vi "Play Editor.vi"() -> ()   [LabVIEW 2015]
uses:
  Autonomous VIs/Autonomous Exec/Autonomous Play Definition.ctl
  Autonomous VIs/Autonomous Commands/Autonomous Command Names.ctl
  <vilib>/FTP/NI_FTP.lvlib
panel:
  in  "Connect\nto Robot":bool
  in  "Reload Folder":bool
  out "Error \nSending \nFiles":errorcluster
  out "Error \nRetrieving \nFiles":errorcluster
  in  "Empty Play Definition":T1 caption="Play"
  in  "Robot IP Address":string(combo)="10.xx.yy.2"
  in  "Download Plays":bool
  in  "Connected to Robot":bool
  in  "Send Plays":bool
  out "Create Play Error":errorcluster
  out "Play Read Error":errorcluster
  in  "Static Form":bool
  out "Commit Play Error":errorcluster
  in  "Current File Refnum":refnum<file>
  in  "Is a File":bool
  in  "Commit Play Changes":bool
  in  "Auto Directory":path
  in  "Finish":bool
  in  "Current Directory":path
  in  "Create New Play":bool
  in  "Play Selector Box":string(combo)
  in  "Play Currently Open":T1 caption="Play"
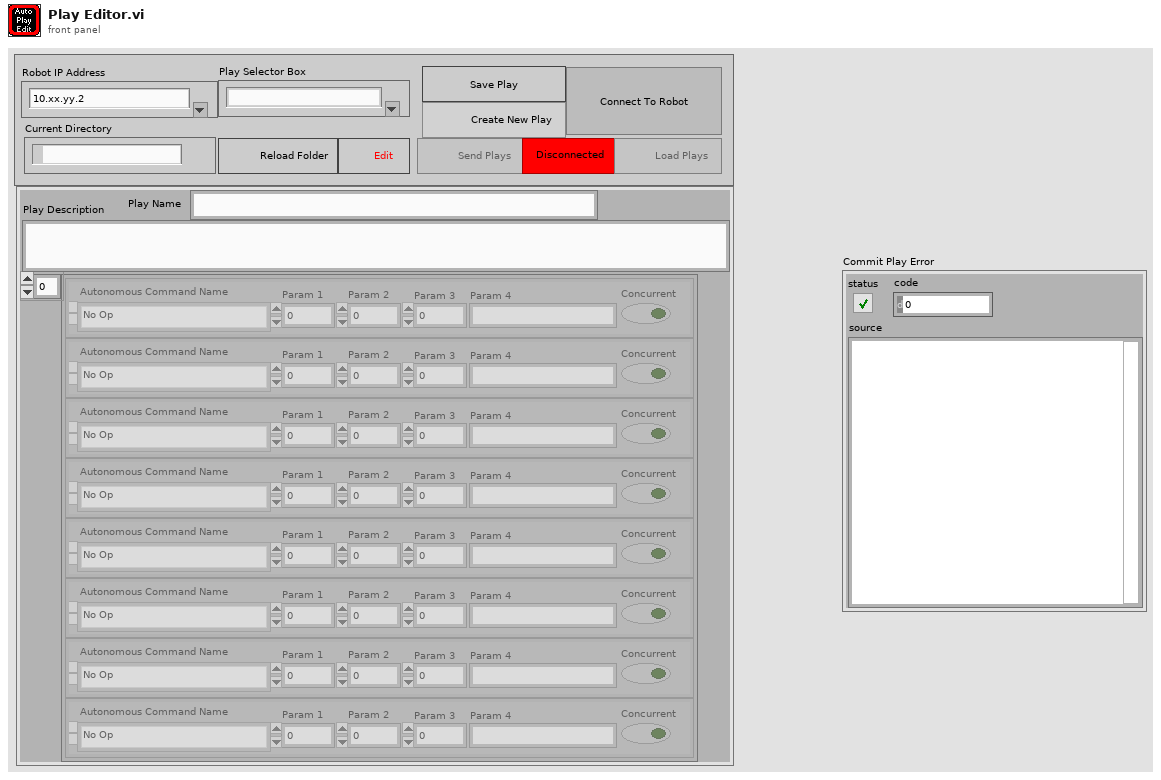
[diagram p1: front panel]
types:
  T1 = typedef "Autonomous Play Definition.ctl" = cluster{"Play Name":string, "Command List":cluster{"Param 1":dbl, "Param 2":dbl, "Autonomous Command Name":T2, "Concurrent":bool, "Param 3":dbl, "Param 4":string}[], "Play Description":string}
  T2 = typedef "Autonomous Command Names.ctl" = enum16{"No Op", "Drive Time", "Run Motion Profile", "Turn to Heading", "Turn To Target", "Cross Defense", "Fire", "Wait", "Reset Gyro", "Grabber Setpoints", "Manual Grabber", "Roller", "Autorange Command", "Reposition"}
  T3 = typedef "NI_FTP.lvlib/FTP Session.ctl" = refnum<k5>
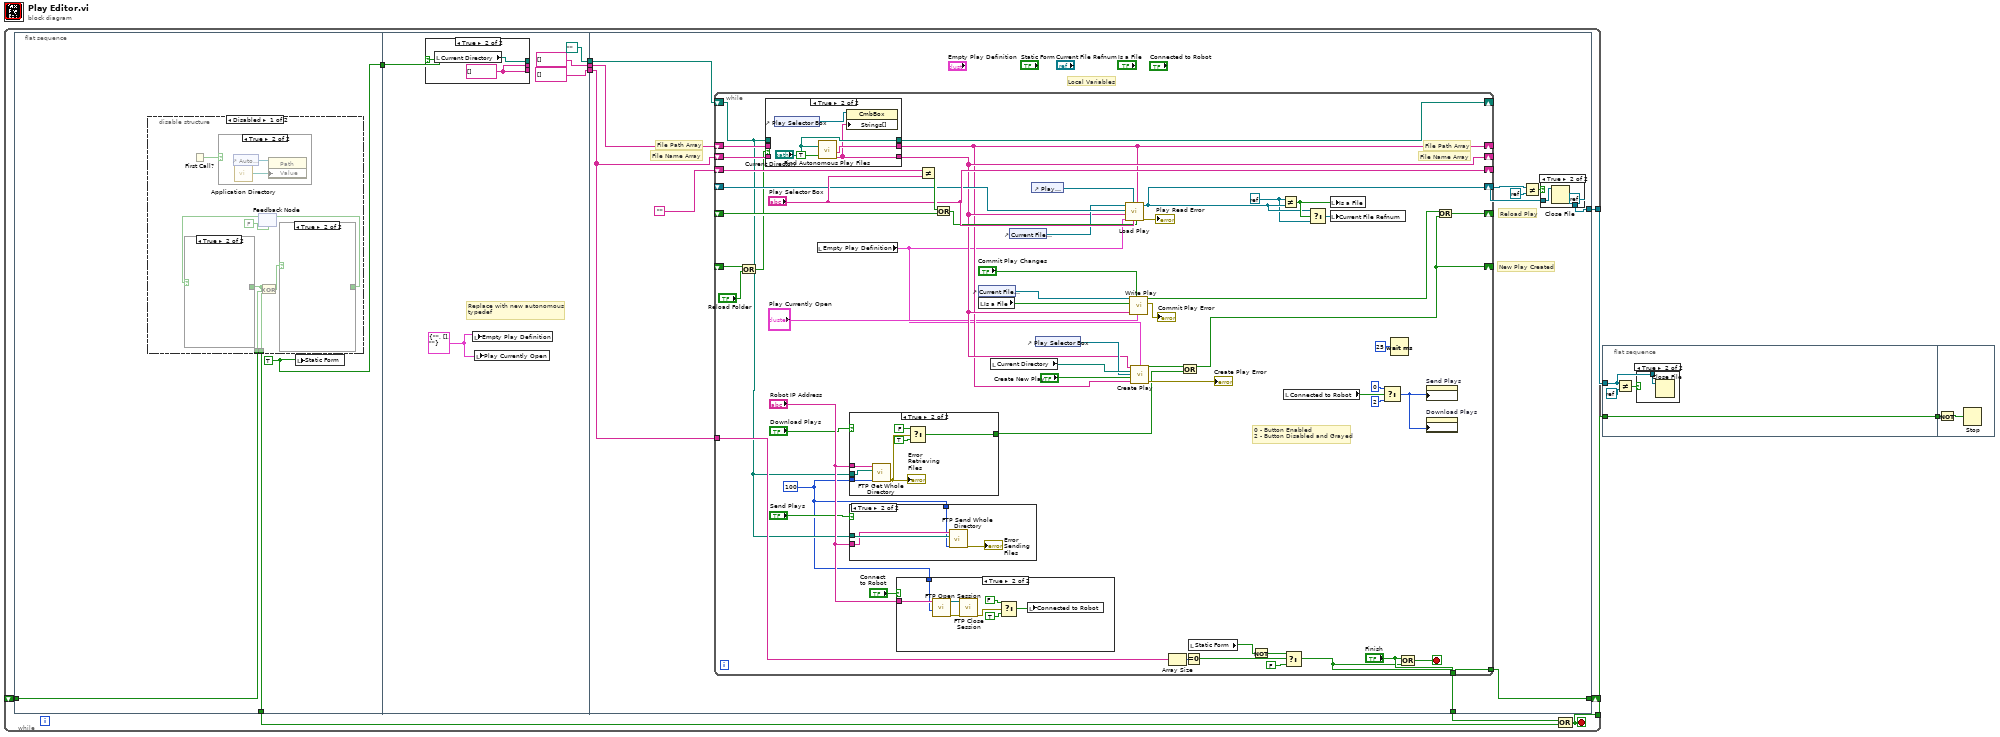
[diagram p0: block diagram]
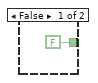
[diagram p3: hidden frame]
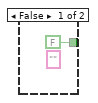
[diagram p4: hidden frame]
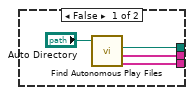
[diagram p7: hidden frame]
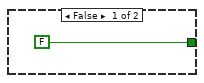
[diagram p11: hidden frame]
diagram:
  n1 = while {
    shift-right: [w10] -> _
    shift-left: _ -> [w9]
    tunnel: [w7] -> w2
    tunnel: [w6] -> w1
    stop <- w7 stop-if-true
    n2 = flat-sequence {
      tunnel: [w15] -> w8
      tunnel: w9 -> [w16]
      tunnel: [w14] -> w4
      tunnel: [string[] [] ("Filepath Array")] -> w13
      tunnel: [path "" ("Current Directory")] -> w12
      tunnel: [string[] [] ("Filepath Array")] -> w5
      tunnel: w4 -> [w32]
      tunnel: w13 -> [w40]
      tunnel: w12 -> [w39]
      tunnel: [w47] -> w11
      tunnel: [w44] -> w10
      tunnel: [w41] -> w6
      tunnel: w5 -> [w42]
      frame #0 {
        w14 = TRUE ("Static Form")
        n3 = disable-structure shown="Disabled" {
          disable-tunnel: w16 -> [w22 _]
          disable-tunnel: [w17 _] -> w15
          frame Disabled {
            n4 = First Call?() -> (First Call?: T/F=w23:bool)
            n5 = case shown="True" w23 {
              frame False {
              }
              frame True {
                n6 = control-ref of="Auto Directory"() -> (w27:refnum<vi>)
                n7 = call <vilib>:"Application Directory.vi"() -> ("Application Directory"=w26:path)
                n8 = property class="Path"(reference=w27, "Value"=w26) -> ()  [unwired: 1 in, 2 out]
              }
            }
            n9 = feedback #1(FALSE ("OK")) -> (w19:bool)
            n10 = case shown="True" w19 {
              tunnel: [FALSE ("No") _] -> w17
              frame False {
              }
              frame True {
              }
            }
            n11 = Exclusive Or(1:w22, 2:w17) -> (0:w21:bool)
            n12 = case shown="True" w21 {
              tunnel: [FALSE ("OK") _] -> w20
              frame False {
                (unwired) "" ("Full Directory")
              }
              frame True {
              }
            }
            n13 = feedback-in #1(w20) -> ()
          }
          frame Enabled {
          }
        }
        n14 = local write "Static Form"(w14) -> ()
      }
      frame #1 {
        w31 = T1 {"Play Name"="", "Command List"=[], "Play Description"=""} ("Play 1")
        # "Replace with new autonomous\ntypedef"
        n15 = case shown="True" w32 {
          tunnel: [w35 w37] -> _
          tunnel: [w34 w38] -> _
          tunnel: [w33 w38] -> _
          frame False {
            n16 = call "Find Autonomous Play Files.vi"("Application Directory"="Auto Directory") -> ("Application Directory"=w35:path, "Filepath Array"=w33:string[], "filename array"=w34:string[])  [unwired: 2 in, 1 out]
          }
          frame True {
            w38 = string[] [] ("Filepath Array")
            n17 = local read "Current Directory"() -> (w37:path)
          }
        }
        n18 = local write "Empty Play Definition"(w31) -> ()
        n19 = local write "Play Currently Open"(w31) -> ()
      }
      frame #2 {
        # "Local Variables"
        # "File Path Array"
        # "File Name Array"
        # "New Play Created"
        # "Reload Play"
        n20 = while {
          shift-right: ["Play Selector Box"] -> _
          shift-left: "" -> [w107]
          shift-right: [w98] -> w43
          shift-left: _ -> [w104]
          shift-right: [w82] -> _
          shift-left: _ -> [w94]
          tunnel: w40 -> [w102]
          tunnel: ["Finish"] -> w47
          tunnel: [w87] -> w44
          shift-right: [w60] -> _
          shift-left: _ -> [w57]
          shift-right: [w72] -> _
          shift-left: w42 -> [w84]
          shift-right: [w73] -> _
          shift-left: w40 -> [w83]
          shift-right: [w55] -> _
          shift-left: w39 -> [w54]
          stop <- w103 stop-if-true
          w53 = 100 ("timeout ms (60000)")
          w96 = refnum<k0> refnum
          # "0 - Button Enabled\n2 - Button Disabled and Grayed"
          # "File Path Array"
          # "File Name Array"
          n21 = Or(x=w57, y="Reload Folder") -> (x .or. y?=w58:bool)
          n22 = case shown="True" w58 {
            tunnel: [w130 w135] -> w72
            tunnel: [w129 w131] -> w73
            tunnel: w84 -> [w130 _]
            tunnel: w83 -> [w129 _]
            tunnel: w54 -> [w128 _]
            tunnel: [w128 "Current Directory"] -> w55
            frame False {
            }
            frame True {
              n23 = control-ref of="Play Selector Box"() -> (w132:refnum<vi>)
              n24 = call "Find Autonomous Play Files.vi"("Application Directory"="Current Directory", "Do not include file\nsuffix"=TRUE ("Do not include\nstring ending")) -> ("Filepath Array"=w135:string[], "filename array"=w131:string[])  [unwired: 1 in, 2 out]
              n25 = property class="CmbBox"(reference=w132, "Strings[]"=w131) -> ()  [unwired: 1 in, 2 out]
            }
          }
          n26 = local read "Empty Play Definition"() -> (w64:T1)
          n27 = case shown="True" "Download Plays" {
            tunnel: w54 -> [_ w127]
            tunnel: "Robot IP Address" -> [_ w126]
            tunnel: [FALSE ("Load New Play") w122] -> w59
            tunnel: w53 -> [_ w121]
            frame False {
            }
            frame True {
              n28 = call "FTP Get Whole Directory.vi"("timeout ms (60000)"=w121, "Local Folder of Autonomous Plays"=w127, "host"=w126) -> ("error out"=w125:errorcluster)  [unwired: 8 in]
              "Error \nRetrieving \nFiles" <- w125
              n29 = Select(t=FALSE, s=w125, f=TRUE ("Load New Play")) -> (s? t:f=w122:bool)
            }
          }
          n30 = case shown="True" "Send Plays" {
            tunnel: w54 -> [_ w119]
            tunnel: "Robot IP Address" -> [_ w118]
            tunnel: w53 -> [_ w116]
            frame False {
            }
            frame True {
              n31 = call "FTP Send Whole Directory.vi"("timeout ms (60000)"=w116, "Local Folder of Autonomous Plays"=w119, "host"=w118) -> ("error out"=→"Error \nSending \nFiles":errorcluster)  [unwired: 8 in]
            }
          }
          n32 = case shown="True" "Connect\nto Robot" {
            tunnel: "Robot IP Address" -> [_ w115]
            tunnel: w53 -> [_ w108]
            frame False {
            }
            frame True {
              n33 = call <vilib>:"FTP Open Session.vi"("timeout ms (60000)"=w108, "address"=w115) -> ("error out"=w113:errorcluster, "ftp session"=w114:T3)  [unwired: 6 in, 2 out]
              n34 = call <vilib>:"FTP Close Session.vi"("error in (no error)"=w113, "ftp session"=w114) -> ("error out"=w112:errorcluster)  [unwired: 6 in, 3 out]
              n35 = Select(t=FALSE, s=w112, f=TRUE) -> (s? t:f=w109:bool)
              n36 = local write "Connected to Robot"(w109) -> ()
            }
          }
          n37 = Not Equal?(x=w107, y="Play Selector Box") -> (x != y?=w106:bool)
          n38 = Or(x=w106, y=w94) -> (x .or. y?=w90:bool)
          n39 = control-ref of="Current File Refnum"() -> (w77:refnum<vi>)
          n40 = local read "Is a File"() -> (w78:bool)
          n41 = local read "Current Directory"() -> (w76:path)
          n42 = control-ref of="Current File Refnum"() -> (w80:refnum<vi>)
          n43 = control-ref of="Play Currently Open"() -> (w63:refnum<vi>)
          n44 = control-ref of="Play Selector Box"() -> (w75:refnum<vi>)
          n45 = call "Load Play.vi"("Load Play"=w90, "Filepath Array"=w72, "Play Selector Box"="Play Selector Box", "Play Currently Open Property Reference"=w63, "Empty Play Definition"=w64, "filename array"=w73, "Previous Iteration \nFile Refnum"=w104, "Current File Refnum"=w80) -> ("Read file error"=→"Play Read Error":errorcluster, "Output File Refnum"=w98:refnum<file>)  [unwired: 2 in]
          n46 = call "Write Play.vi"("Current Selected Play"="Play Currently Open", "Commit Play Changes"="Commit Play Changes", "filename array"=w73, "Is a File"=w78, "File Refnum"=w77) -> ("File Write Error"=→"Commit Play Error":errorcluster, "Not Cancelled\nLoad File"=w95:bool)  [unwired: 5 in]
          n47 = call "Create Play.vi"("Filename Array in"=w73, "Empty Play Definition"=w64, "Application Directory"=w76, "Play Selection Box Property Reference"=w75, "Create New Play"="Create New Play", "Filepath Array in"=w72) -> ("Load New Play"=w81:bool, "error out"=→"Create Play Error":errorcluster)  [unwired: 6 in, 2 out]
          n48 = Array Size(array=w102) -> (size(s)=w101:i32)
          n49 = Or(x=w81, y=w59) -> (x .or. y?=w60:bool)
          n50 = Equal To 0?(x=w101) -> (x = 0?=w89:bool)
          n51 = local read "Static Form"() -> (w88:bool)
          n52 = Not(x=w88) -> (.not. x?=w86:bool)
          n53 = Not Equal?(x=w96, y=w98) -> (x != y?=w99:bool)
          n54 = local read "Connected to Robot"() -> (w68:bool)
          n55 = Select(t=w86, s=w89, f=FALSE) -> (s? t:f=w87:bool)
          n56 = Select(t=w98, s=w99, f=w96) -> (s? t:f=w97:refnum<file>)
          n57 = local write "Is a File"(w99) -> ()
          n58 = local write "Current File Refnum"(w97) -> ()
          n59 = Select(t=0, s=w68, f=2) -> (s? t:f=w66:i32)
          n60 = Wait (ms)(milliseconds to wait=u32 25) -> ()  [unwired: 1 out]
          n61 = Compound Arithmetic op=OR("Finish", w87) -> (w103:bool)
          n62 = property on="Send Plays" class="Bool"("DisabledEnum"=w66) -> ()  [unwired: 2 in, 2 out]
          n63 = property on="Download Plays" class="Bool"("DisabledEnum"=w66) -> ()  [unwired: 2 in, 2 out]
          n64 = Or(x=w95, y=w60) -> (x .or. y?=w82:bool)
        }
        n65 = Not Equal?(x=w43, y=refnum<k0> refnum) -> (x != y?=w45:bool)
        n66 = case shown="True" w45 {
          tunnel: w43 -> [w49 w51]
          tunnel: [w49 refnum<k0> refnum] -> w41
          frame False {
          }
          frame True {
            n67 = Close File(refnum=w51) -> ()  [unwired: 1 in, 2 out]
          }
        }
      }
    }
    n68 = Compound Arithmetic op=OR(w11, w8) -> (w7:bool)
  }
  n69 = flat-sequence {
    tunnel: [w139] -> w3
    tunnel: w2 -> [w139]
    tunnel: w1 -> [w136]
    tunnel: w3 -> [w142]
    frame #0 {
      n70 = Not Equal?(x=w136, y=refnum<k0> refnum) -> (x != y?=w137:bool)
      n71 = case shown="True" w137 {
        tunnel: w136 -> [_ w140]
        frame False {
        }
        frame True {
          n72 = Close File(refnum=w140) -> ()  [unwired: 1 in, 2 out]
        }
      }
    }
    frame #1 {
      n73 = Not(x=w142) -> (.not. x?=w141:bool)
      n74 = Stop(stop? (T)=w141) -> ()
    }
  }
